vi "Write to Protected Connection.vi"(8 "error in (no error)":errorcluster, 9 "Packet":refnum<class "IPacket.lvclass">, 10 "Connection Writer":refnum<class "ProtectedConnectionWriter.lvclass">, 11 "IWriteStrategy in":refnum<class "IWriteStrategy.lvclass">) -> (0 "error out":errorcluster)   [LabVIEW 2020, in "MessagingInterfaces.lvlib" / "IWriteStrategy.lvclass"]
uses:
  <vilib>/gpm_packages/@cs/Network-interface/Source/MessagingInterfaces/IWriteStrategy/IWriteStrategy.lvclass
  <vilib>/gpm_packages/@cs/Network-interface/Source/ProtectedConnectionWriter/ProtectedConnectionWriter.lvclass
  <vilib>/gpm_packages/@cs/Network-interface/Source/MessagingInterfaces/IPacket/IPacket.lvclass
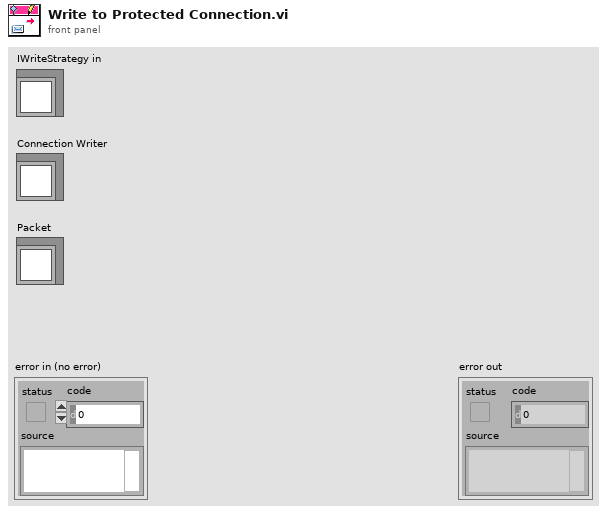
[diagram p1: front panel]
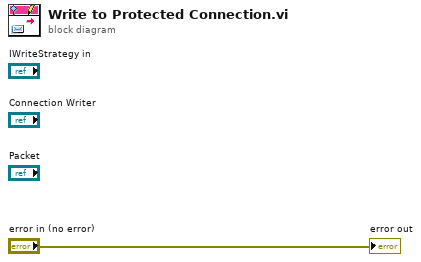
[diagram p0: block diagram]
diagram:
  "error out" <- "error in (no error)"
